vi "Set Units.vi"(8 "error in":errorcluster {"code" format="%.0x"}, 10 "Assign  loss unit according to the chart on the right":dbl=1.0, 11 "VISA resource name":refnum<visa-resource-name>="GPIB12::28::INSTR") -> (0 "error out":errorcluster {"code" format="%.0x"}, 1 "Read out result":string="UC= 9456.092   PF L= 658.76     NS V=0.10   V\r\n", 2 "Send string":string="UNITS 1;\nSHOW UN", 3 "VISA resource name out":refnum<visa-resource-name>)   [LabVIEW 2019, in "AH2500A.lvclass"]
uses:
  AH2500A.lvclass
panel:
  in  "byte count":u32=128
  # "Set the lossunit"
  # "Default setting is 1"
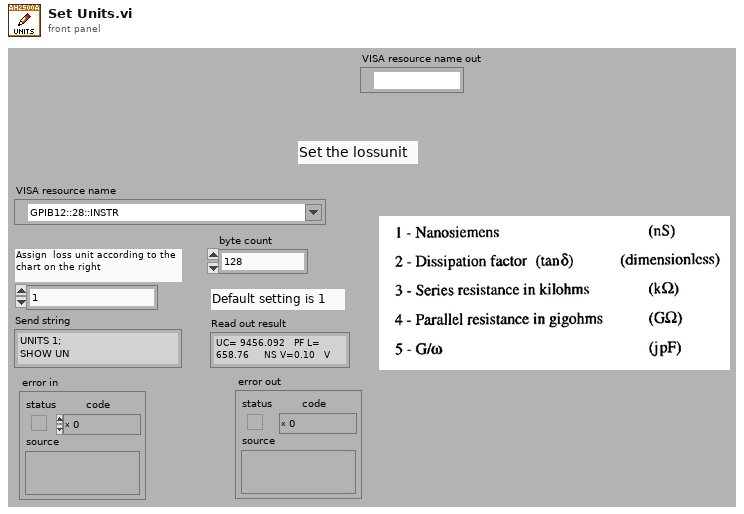
[diagram p1: front panel]
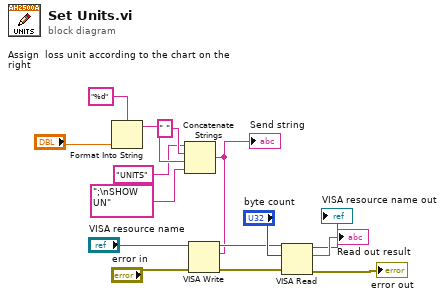
[diagram p0: block diagram]
diagram:
  n1 = Format Into String(format string="%d", "Assign  loss unit according to the chart on the right") -> (resulting string=w11:string)  [unwired: 2 in, 1 out]
  n2 = Concatenate Strings("UNITS" ("string"), " " ("string"), w11, ";\nSHOW UN" ("format string")) -> (w4:string)
  "Send string" <- w4
  n3 = VISA Write(VISA resource name="VISA resource name", write buffer=w4, error in (no error)="error in") -> (VISA resource name out=w7:refnum<visa-resource-name>, error out=w6:errorcluster)  [unwired: 1 out]
  n4 = VISA Read(VISA resource name=w7, byte count="byte count", error in (no error)=w6) -> (VISA resource name out=→"VISA resource name out":refnum<visa-resource-name>, read buffer=→"Read out result":string, error out=→"error out":errorcluster)  [unwired: 1 out]
